vi "follow.vi"() -> ()   [LabVIEW 2020]
uses:
  Classes/Config/Config.lvclass
  Classes/Detector/UV-VIS_AVANTES/UV-VIS_AVANTES.lvclass
  C:/dev/TRANCON/Classes/GeneralFunctionality/GeneralFunctionality.lvclass
  Classes/GeneralFunctionality/GeneralFunctionality.lvclass/GeneralFunctionality.ctl
  dependecies/average-2Darray-SD_double.vi
  <vilib>/Utility/file.llb/Read Delimited Spreadsheet (DBL).vi
  Classes/GeneralFunctionality/GeneralFunctionality.lvclass
  <vilib>/Analysis/NI_AALPro.lvlib
panel:
  in  "TRABS":bool
  in  "convert":bool
  in  "to_":i32
  in  "from_":i32
  out "Waves":dbl[](array[numeric])
  out "Time":dbl[](array[numeric])
  in  "load":bool
  out "DATA":dbl[][](graph)
  in  "wave":dbl
  out "kinetics":T1(graph)
  out "spectrum":T1(graph)
  out "diff, min":dbl
  out "diff, sec":dbl
  out "current time":timestamp
  out "start time":timestamp
  in  "set zero":bool
  out "start":bool
  out "#":i32
  in  "total points":i32=100
  in  "file (use dialog)":path=path "C:/Users/Sergey Denisov/Desktop/test.txt"
  in  "save":bool
  in  "average":i32=10 min=1
  in  "wait, s":dbl=1.0
  in  "Read":bool
  in  "stop":bool
  in  "Path":path=path "C:/Users/Sergey Denisov/Documents/REPS/TRANCON/settings/settingsDetector.ini"
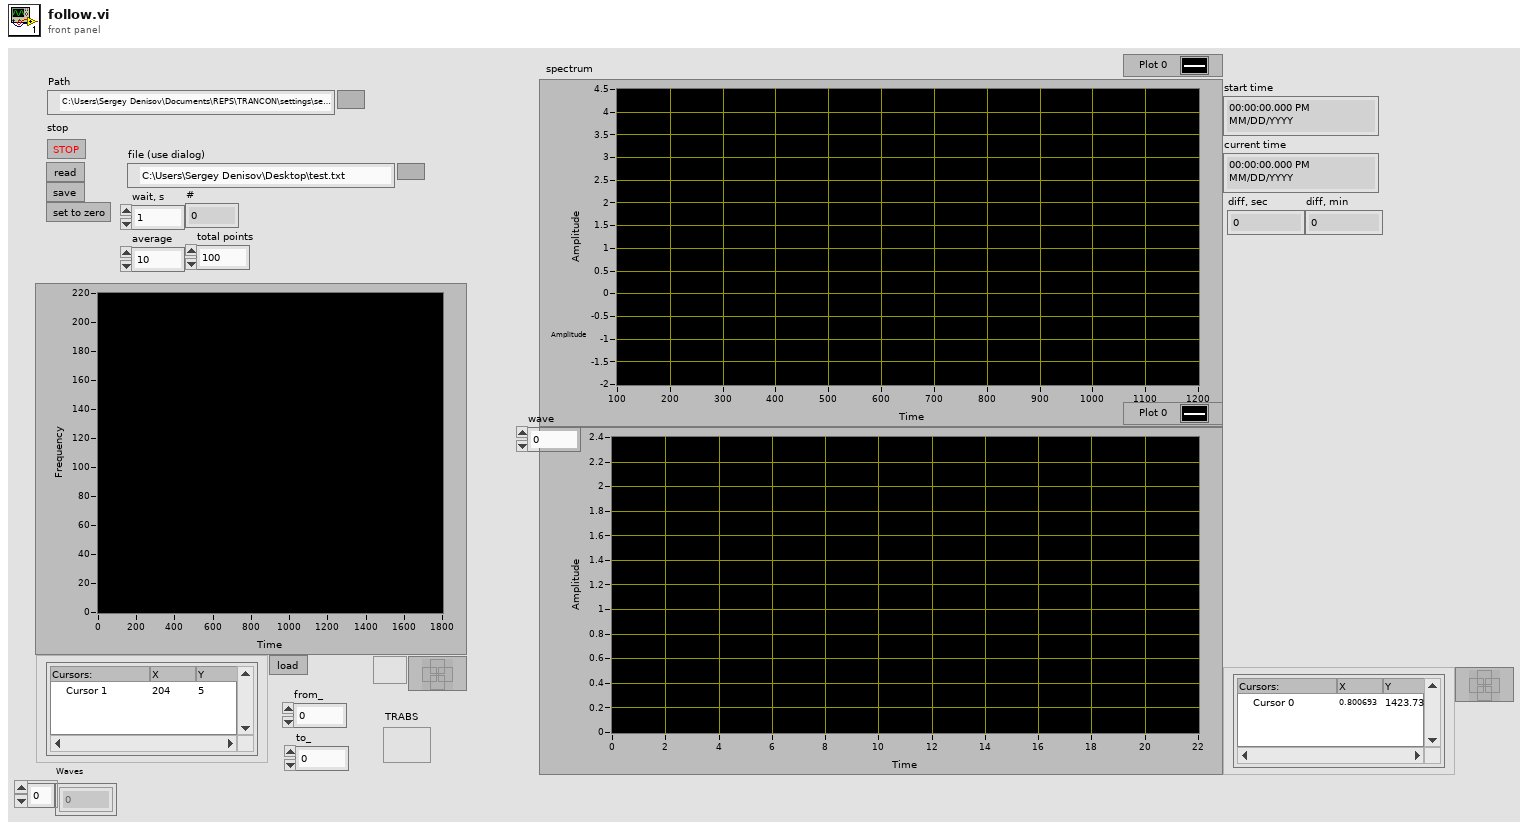
[diagram p1: front panel]
types:
  T1 = cluster{"a_pWaveLength":dbl[], "out array":dbl[]}
  T2 = typedef "LVDateTimeRec.ctl" = cluster{"fractional second":dbl, "second":i32, "minute":i32, "hour":i32, "day of month":i32, "month":i32, "year":i32, "day of week":i32, "day of year":i32, "DST":i32}
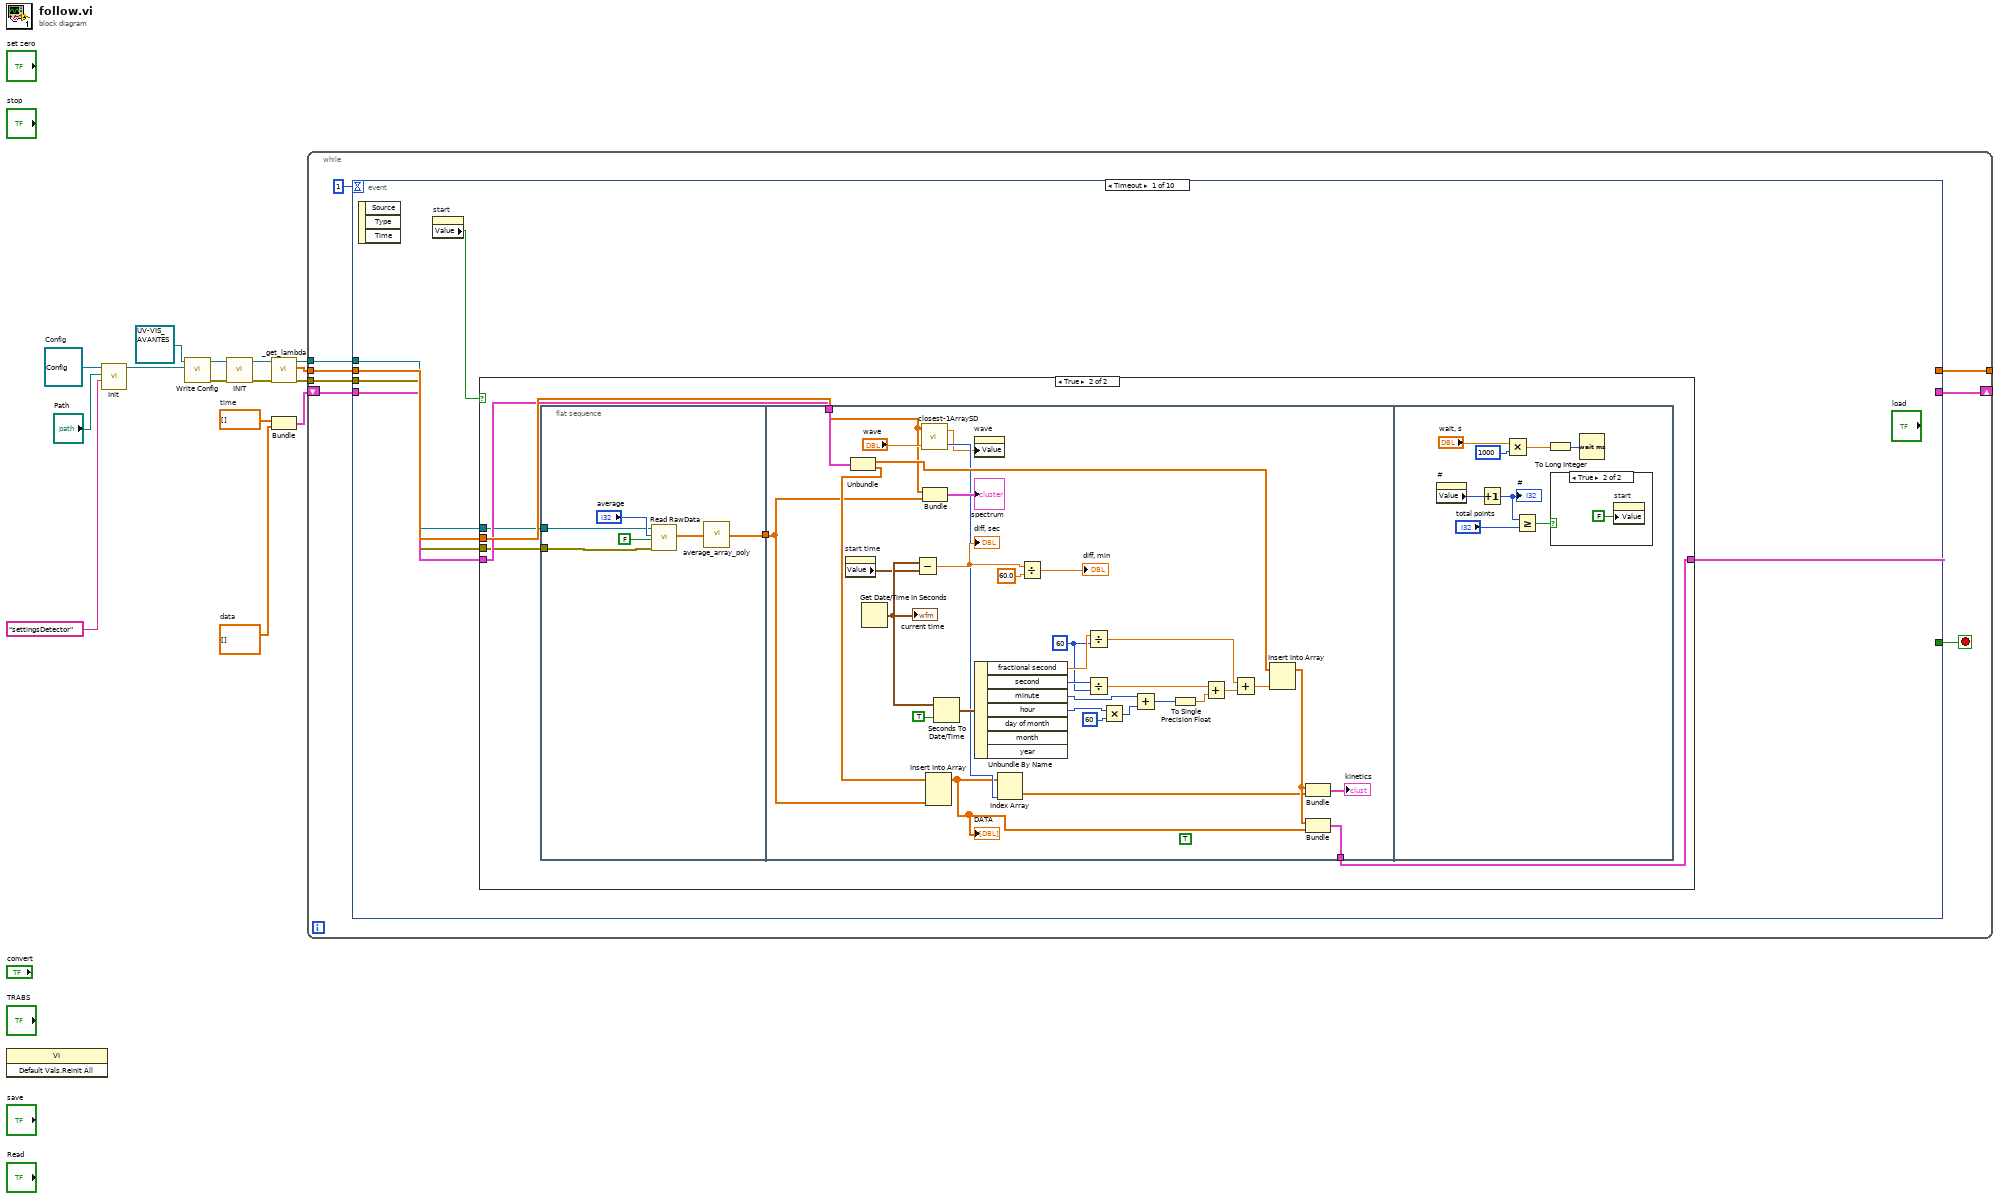
[diagram p0: block diagram]
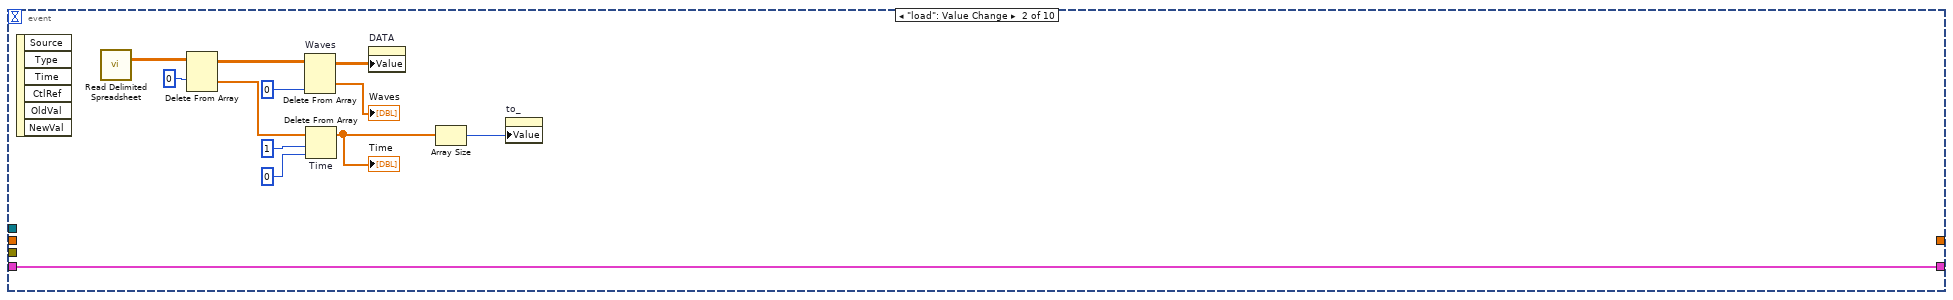
[diagram p4: hidden frame]
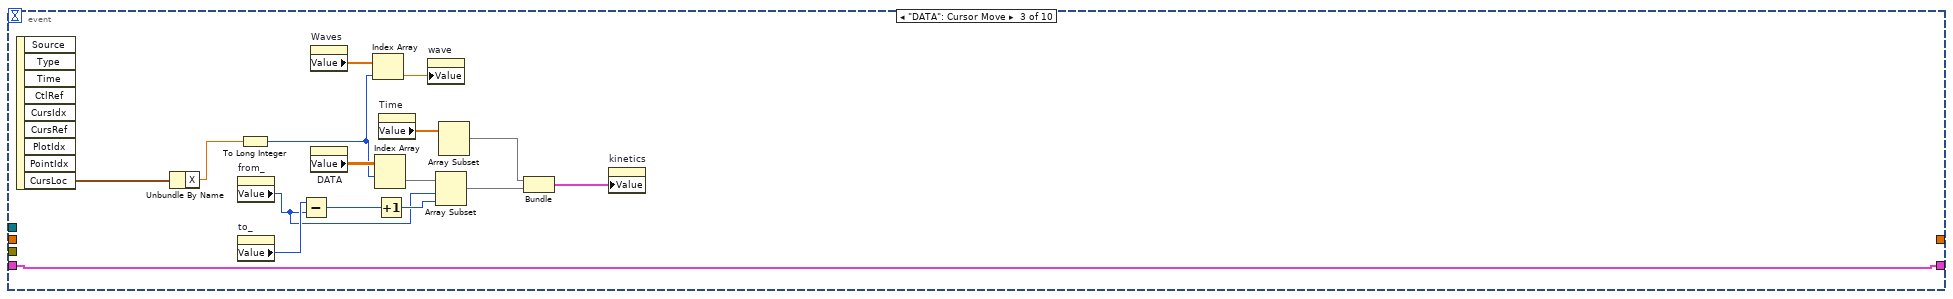
[diagram p5: hidden frame]
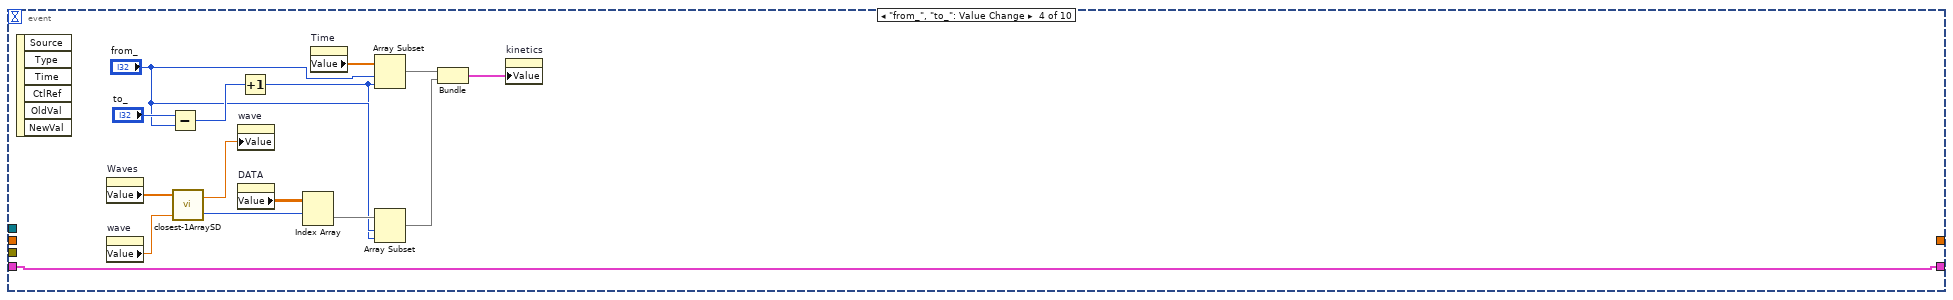
[diagram p6: hidden frame]
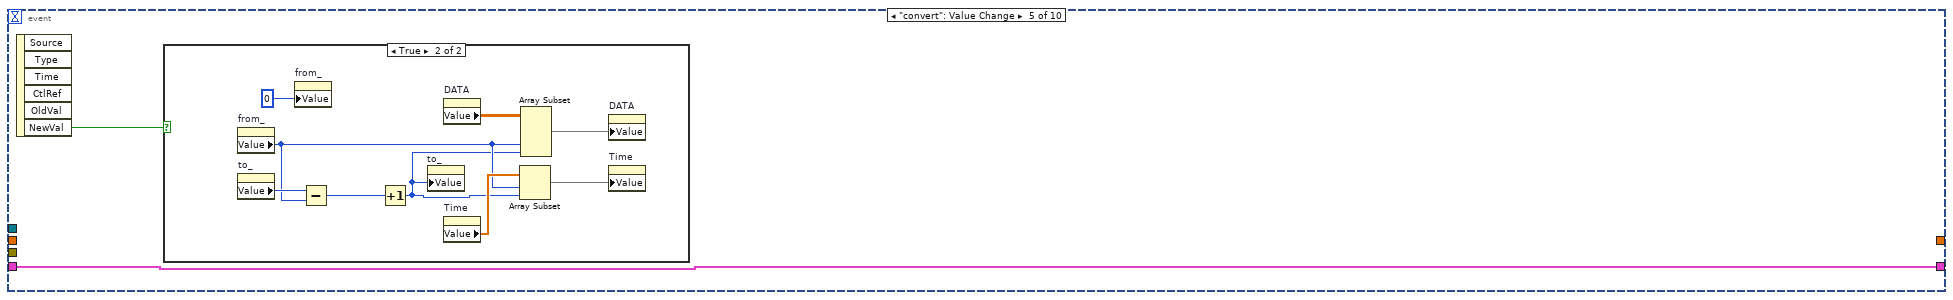
[diagram p7: hidden frame]
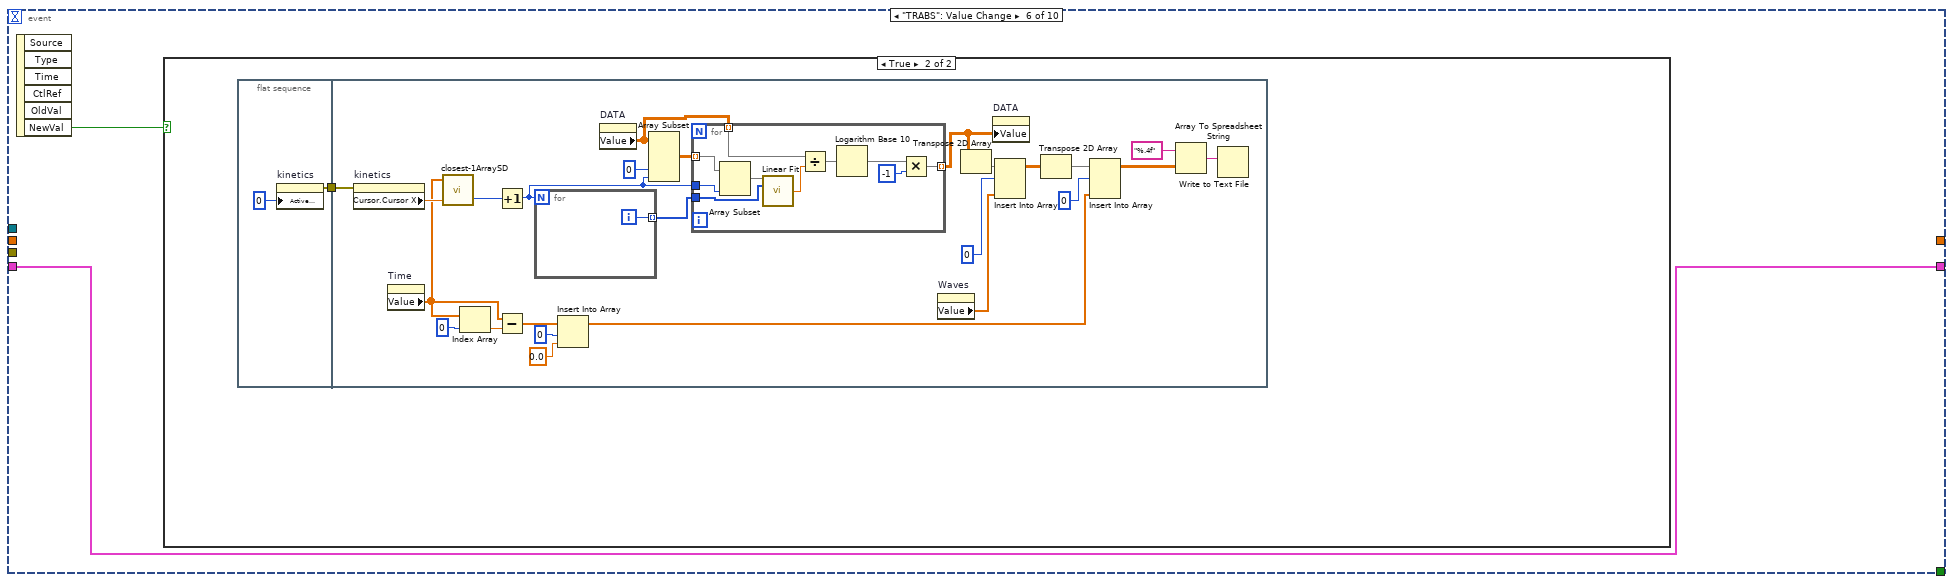
[diagram p9: hidden frame]
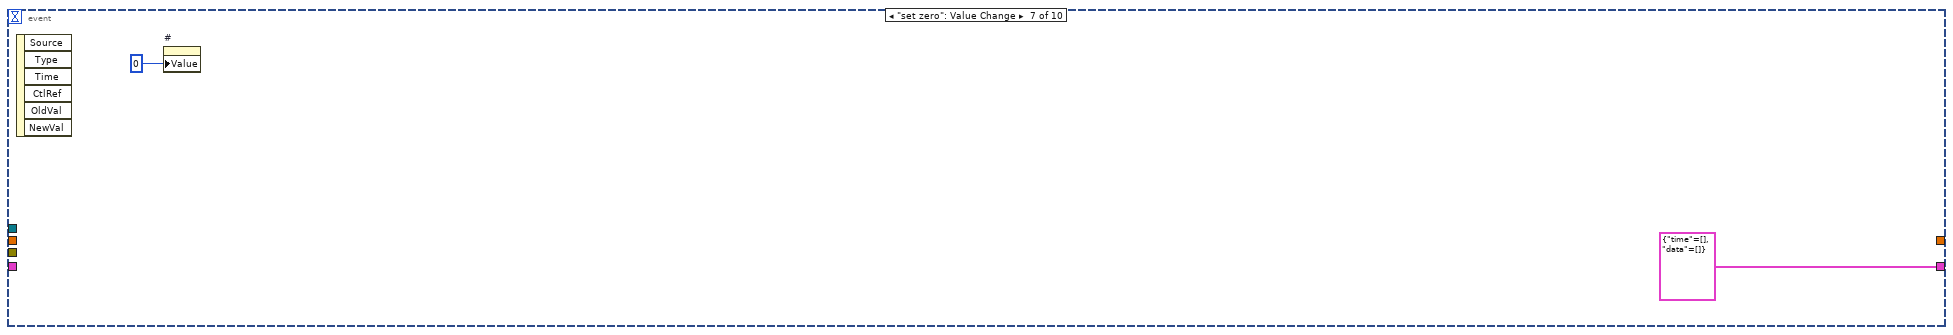
[diagram p11: hidden frame]
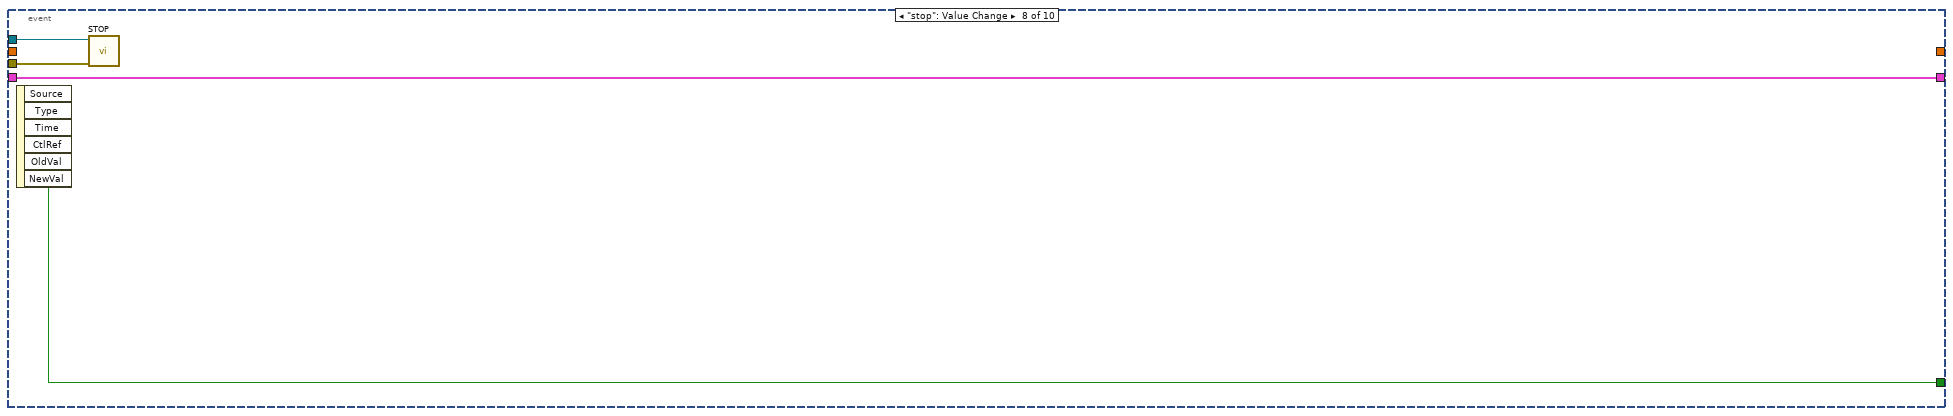
[diagram p12: hidden frame]
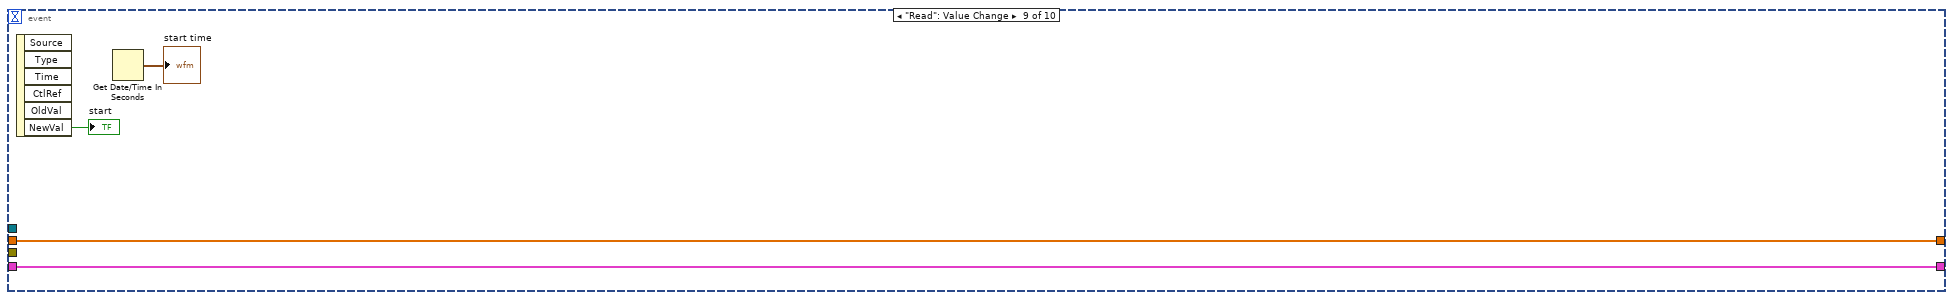
[diagram p13: hidden frame]
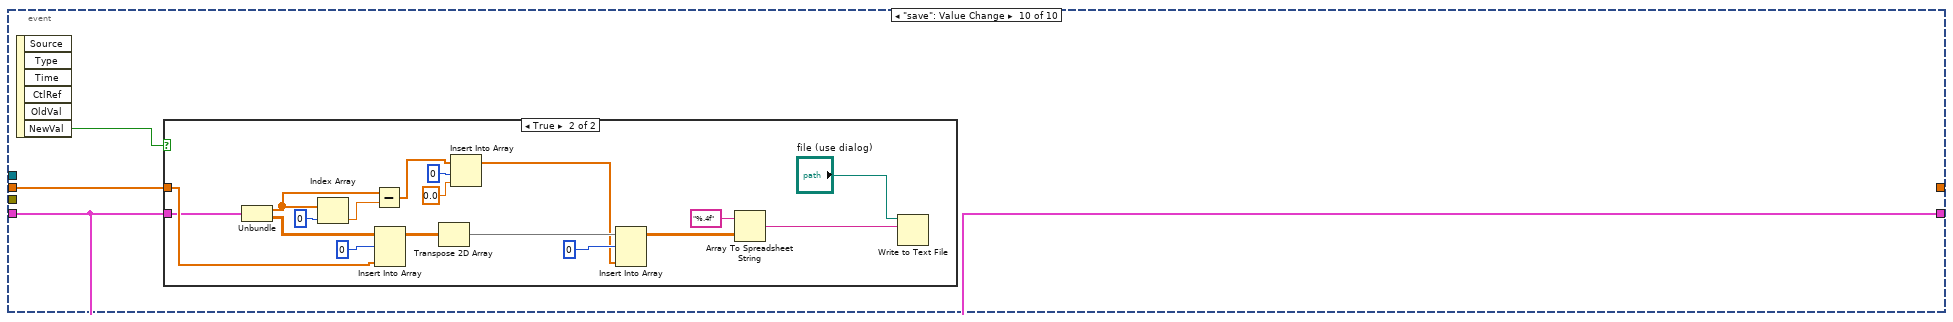
[diagram p14: hidden frame]
diagram:
  w1 = dbl[] []  # time
  w3 = dbl[][] []  # data
  w15 = refnum<class "Config.lvclass"> refnum  # Config
  n1 = invoke class="VI" method="Default Vals.Reinit All"() -> ()  [unwired: 3 in, 3 out]
  n2 = call "Init.vi"("Name"="settingsDetector", "Path"="Path", "Config in"=w15) -> ("Config out"=w11:refnum<class "Config.lvclass">)  [unwired: 7 in, 1 out]
  n3 = call "Write Config.vi"("Config.lvclass"=w11, "GeneralFunctionality en entrée"=refnum<class "UV-VIS_AVANTES.lvclass"> refnum ("UV-VIS_AVANTES in")) -> ("error out"=w9:errorcluster, "GeneralFunctionality en sortie"=w10:refnum<class "UV-VIS_AVANTES.lvclass">)  [unwired: 8 in]
  n4 = call-dynamic "INIT.vi"("error in (no error)"=w9, "UV-VIS_AVANTES in"=w10) -> ("error out"=w8:errorcluster, "UV-VIS_AVANTES out"=w7:refnum<class "UV-VIS_AVANTES.lvclass">)  [unwired: 8 in]
  n5 = call "_get_lambda.vi"("error in (no error)"=w8, "UV-VIS_AVANTES in"=w7) -> ("error out"=w5:errorcluster, "a_pWaveLength"=w4:dbl[], "UV-VIS_AVANTES out"=w6:refnum<class "UV-VIS_AVANTES.lvclass">)  [unwired: 7 in]
  n6 = Bundle("time"=w1, "data"=w3) -> (w2:cluster{"time":dbl[], "data":dbl[][]})  [unwired: 1 in]
  n7 = while {
    tunnel: w5 -> [w21]
    tunnel: w6 -> [w20]
    tunnel: w4 -> [w18]
    shift-right: [w16] -> _
    shift-left: w2 -> [w19]
    tunnel: [w17] -> _
    stop <- w22 stop-if-true
    n8 = event shown="[0] Timeout" {
      selector: _ -> [_ _ _ _ _ _ _ _ _ _]
      dyn-events: _ -> [_ _ _ _ _ _ _ _ _ _]
      timeout: 1 -> [_ _ _ _ _ _ _ _ _ _]
      tunnel: [_ _ _ _ _ _ _ w186 _ _] -> w22
      tunnel: w21 -> [w25 _ _ _ _ _ _ w185 _ _]
      tunnel: w20 -> [w26 _ _ _ _ _ _ w184 _ _]
      tunnel: w19 -> [w27 w97 w113 w114 w129 w140 _ w183 w190 w192]
      tunnel: w18 -> [w28 _ _ _ _ _ _ _ w189 w193]
      tunnel: [w24 w97 w113 w114 w129 w140 cluster{"time":dbl[], "data":dbl[][]} {"time"=[], "data"=[]} w183 w190 w192] -> w16
      tunnel: [_ _ _ _ _ _ _ _ w189 _] -> w17
      event Timeout {
        n9 = event-data() -> ()  [unwired: 1 in, 3 out]
        n10 = property on="start" class="Bool (strict)"() -> ("Value"=w29:bool)  [unwired: 2 in, 2 out]
        n11 = case shown="True" w29 {
          tunnel: w28 -> [_ w35]
          tunnel: w27 -> [w30 w34]
          tunnel: w26 -> [_ w33]
          tunnel: w25 -> [_ w32]
          tunnel: [w30 w31] -> w24
          frame False {
          }
          frame True {
            n12 = flat-sequence {
              tunnel: [w39] -> w36
              tunnel: w33 -> [w38]
              tunnel: w32 -> [w37]
              tunnel: w36 -> [w73]
              tunnel: [w74] -> w31
              tunnel: w35 -> [w46]
              tunnel: w34 -> [w71]
              frame #0 {
                n13 = call-dynamic "Read RawData.vi"("error in (no error)"=w37, "WCM_max_value"=FALSE, "# of scans"="average", "UV-VIS_AVANTES in"=w38) -> ("Channel I"=w41:sgl[][])  [unwired: 3 in, 4 out]
                n14 = call-poly "average_array_poly.vi"("2D array"=w41) -> ("out array"=w39:dbl[])
              }
              frame #1 {
                w59 = 60 ("y")
                (unwired) TRUE ("want seconds? (F)")
                n15 = property on="start time" class="AbsTime (strict)"() -> ("Value"=w54:timestamp)  [unwired: 2 in, 2 out]
                n16 = Unbundle(w71) -> ("time"=w75:dbl[], "data"=w76:dbl[][])
                n17 = Get Date/Time In Seconds() -> (seconds since 1Jan1904=w55:timestamp)
                "current time" <- w55
                n18 = Subtract(x=w55, y=w54) -> (x-y=w53:dbl)
                "diff, sec" <- w53
                n19 = call "closest-1ArraySD.vi"("desired element"="wave", "1D Array"=w46) -> ("closest index"=w45:i32, "closest element"=w44:dbl)  [unwired: 1 in]
                n20 = Bundle("a_pWaveLength"=w46, "out array"=w73) -> (→"spectrum":T1)  [unwired: 1 in]
                n21 = Insert Into Array(array=w76, new element=w73) -> (w43:dbl[][])  [unwired: 2 in]
                "DATA" <- w43
                n22 = Seconds To Date/Time(time stamp (now)=w55, to UTC (F)=TRUE) -> (date time rec=w63:T2)
                n23 = property on="wave" class="DigNum (strict)"("Value"=w44) -> ()  [unwired: 2 in, 2 out]
                n24 = Unbundle By Name(w63) -> ("fractional second"=w60:dbl, "second"=w67:i32, "minute"=w65:i32, "hour"=w64:i32)  [unwired: 3 out]
                n25 = Index Array(array=w43, index (col)=w45) -> (element=w49:dbl[])  [unwired: 1 in]
                n26 = Divide(x=w53, y=60.0) -> (x/y=→"diff, min":dbl)
                n27 = Divide(x=w60, y=w59) -> (x/y=w58:dbl)
                n28 = Divide(x=w67, y=w59) -> (x/y=w70:dbl)
                n29 = Multiply(x=w64, y=60) -> (x*y=w66:i32)
                n30 = Add(x=w65, y=w66) -> (x+y=w68:i32)
                n31 = To Single Precision Float(number=w68) -> (single precision float=w69:sgl)
                n32 = Add(x=w70, y=w69) -> (x+y=w57:dbl)
                n33 = Add(x=w58, y=w57) -> (x+y=w56:dbl)
                n34 = Insert Into Array(array=w75, new element=w56) -> (w50:dbl[])  [unwired: 1 in]
                n35 = Bundle("time"=w50, "data"=w49) -> (→"kinetics":cluster{"time":dbl[], "data":dbl[]})  [unwired: 1 in]
                n36 = Bundle("time"=w50, "data"=w43) -> (w74:cluster{"time":dbl[], "data":dbl[][]})  [unwired: 1 in]
              }
              frame #2 {
                n37 = property on="#" class="DigNum (strict)"() -> ("Value"=w80:i32)  [unwired: 2 in, 2 out]
                n38 = Increment(x=w80) -> (x+1=w79:i32)
                "#" <- w79
                n39 = Multiply(x="wait, s", y=1000) -> (x*y=w82:dbl)
                n40 = Greater Or Equal?(x=w79, y="total points") -> (x >= y?=w77:bool)
                n41 = To Long Integer(number=w82) -> (32bit integer=w81:i32)
                n42 = case shown="True" w77 {
                  frame False {
                  }
                  frame True {
                    n43 = property on="start" class="Bool (strict)"("Value"=FALSE ("start")) -> ()  [unwired: 2 in, 2 out]
                  }
                }
                n44 = Wait (ms)(milliseconds to wait=w81) -> ()  [unwired: 1 out]
              }
            }
          }
        }
      }
      event "load": Value Change {
        n45 = event-data() -> ()  [unwired: 1 in, 6 out]
        n46 = call-poly <vilib>:"Read Delimited Spreadsheet.vi"() -> ("all rows"=w96:dbl[][])  [unwired: 10 in, 5 out]
        n47 = Delete From Array(array=w96, index (row)=0) -> (deleted portion=w95:dbl[], array with subset deleted=w92:dbl[][])  [unwired: 2 in]
        n48 = Delete From Array "Waves"(array=w92, index (col)=0 ("disabled index (col)")) -> (deleted portion=→"Waves":dbl[], array with subset deleted=w89:dbl[][])  [unwired: 2 in]
        n49 = Delete From Array "Time"(array=w95, length=1, index=0) -> (array with subset deleted=w87:dbl[])  [unwired: 1 out]
        "Time" <- w87
        n50 = property on="DATA" class="IntGraph (strict)"("Value"=w89) -> ()  [unwired: 2 in, 2 out]
        n51 = Array Size(array=w87) -> (size(s)=w86:i32)
        n52 = property on="to_" class="DigNum (strict)"("Value"=w86) -> ()  [unwired: 2 in, 2 out]
      }
      event "DATA": Cursor Move {
        n53 = event-data() -> ("CursLoc"=w112:cluster{"X":dbl, "Y":dbl})  [unwired: 1 in, 8 out]
        n54 = Unbundle By Name(w112) -> ("X"=w111:dbl)
        n55 = property on="from_" class="DigNum (strict)"() -> ("Value"=w100:i32)  [unwired: 2 in, 2 out]
        n56 = property on="to_" class="DigNum (strict)"() -> ("Value"=w105:i32)  [unwired: 2 in, 2 out]
        n57 = To Long Integer(number=w111) -> (32bit integer=w107:i32)
        n58 = Subtract(x=w105, y=w100) -> (x-y=w106:i32)
        n59 = property on="Waves" class="Arr (strict)"() -> ("Value"=w108:dbl[])  [unwired: 2 in, 2 out]
        n60 = property on="DATA" class="IntGraph (strict)"() -> ("Value"=w109:dbl[][])  [unwired: 2 in, 2 out]
        n61 = Index Array(array=w108, index=w107) -> (element=w110:dbl)
        n62 = Index Array(array=w109, index (row)=w107) -> (element=w102:dbl[])  [unwired: 1 in]
        n63 = Increment(x=w106) -> (x+1=w101:i32)
        n64 = property on="Time" class="Arr (strict)"() -> ("Value"=w104:dbl[])  [unwired: 2 in, 2 out]
        n65 = property on="wave" class="DigNum (strict)"("Value"=w110) -> ()  [unwired: 2 in, 2 out]
        n66 = Array Subset(array=w102, index=w100, length=w101) -> (w99:dbl[])
        n67 = Array Subset(array=w104) -> (w103:dbl[])  [unwired: 2 in]
        n68 = Bundle(w103, w99) -> (w98:cluster{dbl[], dbl[]})  [unwired: 1 in]
        n69 = property on="kinetics" class="XYGraph (strict)"("Value"=w98) -> ()  [unwired: 2 in, 2 out]
      }
      event "from_", "to_": Value Change {
        n70 = event-data() -> ()  [unwired: 1 in, 6 out]
        n71 = property on="Waves" class="Arr (strict)"() -> ("Value"=w122:dbl[])  [unwired: 2 in, 2 out]
        n72 = property on="wave" class="DigNum (strict)"() -> ("Value"=w121:dbl)  [unwired: 2 in, 2 out]
        n73 = Subtract(x="to_", y="from_") -> (x-y=w124:i32)
        n74 = call "closest-1ArraySD.vi"("desired element"=w121, "1D Array"=w122) -> ("closest index"=w119:i32, "closest element"=w120:dbl)  [unwired: 1 in]
        n75 = property on="wave" class="DigNum (strict)"("Value"=w120) -> ()  [unwired: 2 in, 2 out]
        n76 = property on="DATA" class="IntGraph (strict)"() -> ("Value"=w128:dbl[][])  [unwired: 2 in, 2 out]
        n77 = Increment(x=w124) -> (x+1=w115:i32)
        n78 = Index Array(array=w128, index (row)=w119) -> (element=w118:dbl[])  [unwired: 1 in]
        n79 = property on="Time" class="Arr (strict)"() -> ("Value"=w126:dbl[])  [unwired: 2 in, 2 out]
        n80 = Array Subset(array=w126, index="from_", length=w115) -> (w123:dbl[])
        n81 = Array Subset(array=w118, index="from_", length=w115) -> (w117:dbl[])
        n82 = Bundle(w123, w117) -> (w127:cluster{dbl[], dbl[]})  [unwired: 1 in]
        n83 = property on="kinetics" class="XYGraph (strict)"("Value"=w127) -> ()  [unwired: 2 in, 2 out]
      }
      event "convert": Value Change {
        n84 = event-data() -> ("NewVal"=w130:bool)  [unwired: 1 in, 5 out]
        n85 = case shown="True" w130 {
          frame False {
          }
          frame True {
            n86 = property on="from_" class="DigNum (strict)"() -> ("Value"=w133:i32)  [unwired: 2 in, 2 out]
            n87 = property on="to_" class="DigNum (strict)"() -> ("Value"=w137:i32)  [unwired: 2 in, 2 out]
            n88 = property on="from_" class="DigNum (strict)"("Value"=0 ("to_")) -> ()  [unwired: 2 in, 2 out]
            n89 = Subtract(x=w137, y=w133) -> (x-y=w136:i32)
            n90 = Increment(x=w136) -> (x+1=w132:i32)
            n91 = property on="to_" class="DigNum (strict)"("Value"=w132) -> ()  [unwired: 2 in, 2 out]
            n92 = property on="DATA" class="IntGraph (strict)"() -> ("Value"=w138:dbl[][])  [unwired: 2 in, 2 out]
            n93 = property on="Time" class="Arr (strict)"() -> ("Value"=w134:dbl[])  [unwired: 2 in, 2 out]
            n94 = Array Subset(array=w134, index=w133, length=w132) -> (w131:dbl[])
            n95 = Array Subset(array=w138, index (col)=w133, length (col)=w132) -> (w135:dbl[][])  [unwired: 2 in]
            n96 = property on="DATA" class="IntGraph (strict)"("Value"=w135) -> ()  [unwired: 2 in, 2 out]
            n97 = property on="Time" class="Arr (strict)"("Value"=w131) -> ()  [unwired: 2 in, 2 out]
          }
        }
      }
      event "TRABS": Value Change {
        n98 = event-data() -> ("NewVal"=w141:bool)  [unwired: 1 in, 5 out]
        n99 = case shown="True" w141 {
          frame False {
          }
          frame True {
            n100 = flat-sequence {
              tunnel: [w143] -> w142
              tunnel: w142 -> [w169]
              frame #0 {
                n101 = property on="kinetics" class="XYGraph (strict)"("Active Cursor"=u32 0) -> (error out=w143:errorcluster)  [unwired: 2 in, 1 out]
              }
              frame #1 {
                n102 = property on="kinetics" class="XYGraph (strict)"(error in=w169) -> ("Cursor.Cursor X"=w168:dbl)  [unwired: 1 in, 2 out]
                n103 = property on="Time" class="Arr (strict)"() -> ("Value"=w148:dbl[])  [unwired: 2 in, 2 out]
                n104 = call "closest-1ArraySD.vi"("desired element"=w168, "1D Array"=w148) -> ("closest index"=w166:i32)  [unwired: 1 in, 1 out]
                n105 = Index Array(array=w148, index=0) -> (element=w151:dbl)
                n106 = Increment(x=w166) -> (x+1=w163:i32)
                n107 = Subtract(x=w148, y=w151) -> (x-y=w150:dbl[])
                n108 = for {
                  N: w163 -> [_]
                  tunnel: [w180] -> w164 mode=indexing
                  i -> [w180]
                }
                n109 = Insert Into Array(array=w150, index=0, new element=0.0 ("new element/subarray")) -> (w154:dbl[])
                n110 = property on="DATA" class="IntGraph (strict)"() -> ("Value"=w145:dbl[][])  [unwired: 2 in, 2 out]
                n111 = Array Subset(array=w145, index (col)=0 ("index"), length (col)=w163) -> (w165:dbl[][])  [unwired: 2 in]
                n112 = for {
                  tunnel: w165 -> [w176] mode=indexing
                  tunnel: w164 -> [w179]
                  tunnel: w163 -> [w178]
                  tunnel: [w172] -> w147 mode=indexing
                  tunnel: w145 -> [w171] mode=indexing
                  n113 = Array Subset(array=w176, length=w178) -> (w177:dbl[])  [unwired: 1 in]
                  n114 = call <vilib>:"Linear Fit.vi"("Y"=w177, "X"=w179) -> ("intercept"=w170:dbl)  [unwired: 9 in, 4 out]
                  n115 = Divide(x=w171, y=w170) -> (x/y=w175:dbl[])
                  n116 = Logarithm Base 10(1:w175) -> (0:w174:dbl[])
                  n117 = Multiply(x=w174, y=-1) -> (x*y=w172:dbl[])
                }
                n118 = property on="Waves" class="Arr (strict)"() -> ("Value"=w149:dbl[])  [unwired: 2 in, 2 out]
                n119 = Transpose 2D Array(2D array=w147) -> (transposed array=w146:dbl[][])
                n120 = property on="DATA" class="IntGraph (strict)"("Value"=w147) -> ()  [unwired: 2 in, 2 out]
                n121 = Insert Into Array(array=w146, index (row)=0, new element=w149) -> (w161:dbl[][])  [unwired: 1 in]
                n122 = Transpose 2D Array(2D array=w161) -> (transposed array=w157:dbl[][])
                n123 = Insert Into Array(array=w157, index (row)=0, new element=w154) -> (w156:dbl[][])  [unwired: 1 in]
                n124 = Array To Spreadsheet String(array=w156, 3:"%.4f" ("format string")) -> (spreadsheet string=w153:string)  [unwired: 1 in]
                n125 = Write to Text File(text=w153) -> ()  [unwired: 3 in, 3 out]
              }
            }
          }
        }
      }
      event "set zero": Value Change {
        n126 = event-data() -> ()  [unwired: 1 in, 6 out]
        n127 = property on="#" class="DigNum (strict)"("Value"=0 ("#")) -> ()  [unwired: 2 in, 2 out]
      }
      event "stop": Value Change {
        n128 = event-data() -> ("NewVal"=w186:bool)  [unwired: 1 in, 5 out]
        n129 = call-dynamic "STOP.vi"("error in (no error)"=w185, "Stop in"=w184) -> ()  [unwired: 8 in, 2 out]
      }
      event "Read": Value Change {
        n130 = event-data() -> ("NewVal"=→"start":bool)  [unwired: 1 in, 5 out]
        n131 = Get Date/Time In Seconds() -> (seconds since 1Jan1904=→"start time":timestamp)
      }
      event "save": Value Change {
        n132 = event-data() -> ("NewVal"=w191:bool)  [unwired: 1 in, 5 out]
        n133 = case shown="True" w191 {
          tunnel: w193 -> [_ w210]
          tunnel: w192 -> [_ w194]
          frame False {
          }
          frame True {
            n134 = Unbundle(w194) -> ("time"=w196:dbl[], "data"=w211:dbl[][])
            n135 = Index Array(array=w196, index=0) -> (element=w197:dbl)
            n136 = Subtract(x=w196, y=w197) -> (x-y=w195:dbl[])
            n137 = Insert Into Array(array=w211, index (row)=0, new element=w210) -> (w208:dbl[][])  [unwired: 1 in]
            n138 = Transpose 2D Array(2D array=w208) -> (transposed array=w203:dbl[][])
            n139 = Insert Into Array(array=w195, index=0, new element=0.0 ("new element/subarray")) -> (w200:dbl[])
            n140 = Insert Into Array(array=w203, index (row)=0, new element=w200) -> (w202:dbl[][])  [unwired: 1 in]
            n141 = Array To Spreadsheet String(array=w202, 3:"%.4f" ("format string")) -> (spreadsheet string=w199:string)  [unwired: 1 in]
            n142 = Write to Text File(file (use dialog)="file (use dialog)", text=w199) -> ()  [unwired: 2 in, 3 out]
          }
        }
      }
    }
  }
